vi "Get Status.vi"(8 "error in (no error)":errorcluster, 11 "IObject in":refnum<class "IObject.lvclass">) -> (0 "error out":errorcluster, 2 "Status":string, 3 "IObject out":refnum<class "IObject.lvclass">)   [LabVIEW 2013, in "IObject.lvclass"]
uses:
  IObject.lvclass
  IObject.lvclass/IObject.ctl
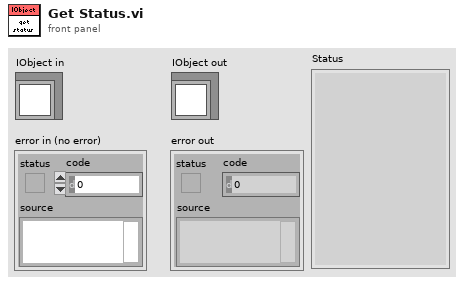
[diagram p1: front panel]
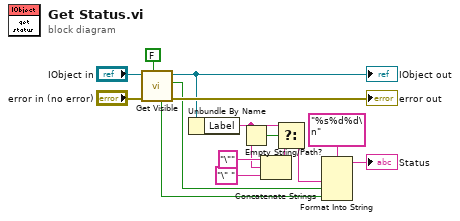
[diagram p0: block diagram]
diagram:
  n1 = call-dynamic "Get Visible.vi"("Hide if children are hidden? [T]"=FALSE, "error in (no error)"="error in (no error)", "IObject in"="IObject in") -> ("error out"=→"error out":errorcluster, "Visible?"=w12:bool, "IObject out"=w10:refnum<class "IObject.lvclass">, "Item visible?"=w11:bool)  [unwired: 5 in]
  "IObject out" <- w10
  n2 = Unbundle By Name(w10) -> ("Label"=w4:string)
  n3 = Empty String/Path?(string/path=w4) -> (empty?=w5:bool)
  n4 = Concatenate Strings("\"" ("string"), w4, "\" " ("string")) -> (w3:string)
  n5 = Select(t=w4, s=w5, f=w3) -> (s? t:f=w2:string)
  n6 = Format Into String(format string="%s%d%d\n", w2, w12, w11) -> (resulting string=→"Status":string)  [unwired: 2 in, 1 out]
